vi "Build Delete.vi"(8 "error in (no error)":errorcluster, 9 "tableName":string, 10 "DynamicParameters in":refnum<class "DynamicParameters.lvclass">, 11 "DbConnection in":refnum<class "DbConnection.lvclass">) -> (0 "error out":errorcluster, 2 "Query":string, 3 "DbConnection out":refnum<class "DbConnection.lvclass">)   [LabVIEW 2020, in "ORM.lvlib" / "DbConnection.lvclass"]
uses:
  DbConnection.lvclass
  DynamicParameters/DynamicParameters.lvclass
  DbConnection.lvclass/DbConnection.ctl
  DynamicParameters/DynamicParameters.lvclass/DynamicParameters.ctl
  Read ColumnNameEqualsValueFormat.vi
  DynamicParameters/Read FieldNames.vi
  DynamicParameters/Read ParameterNames.vi
  DynamicParameters/Read KeyProperties.vi
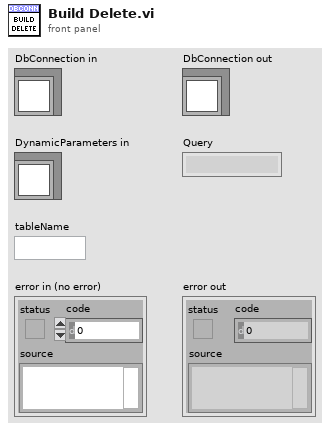
[diagram p1: front panel]
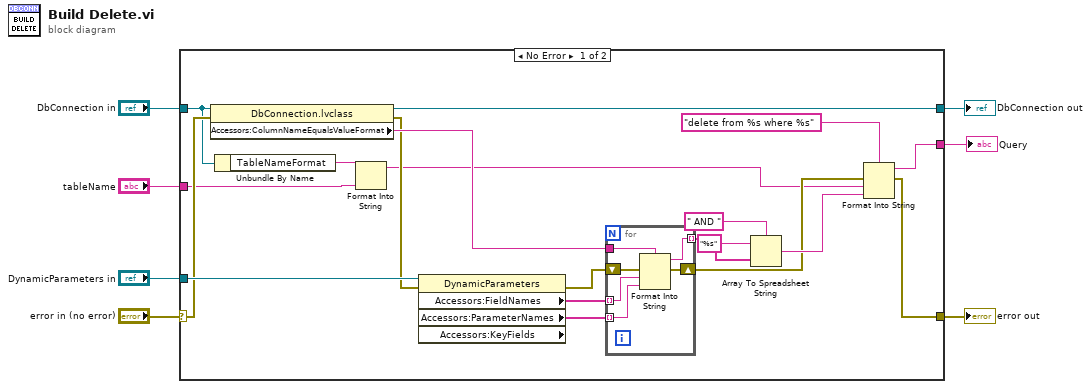
[diagram p0: block diagram]
diagram:
  n1 = case shown="No Error" "error in (no error)" {
    selector: "error in (no error)" -> [w18 w35]
    tunnel: [w14 w35] -> w6
    tunnel: [w27 w34] -> w4
    tunnel: "DbConnection in" -> [w11 w34]
    tunnel: "DynamicParameters in" -> [w26 _]
    tunnel: "tableName" -> [w9 _]
    tunnel: [w19 _] -> w1
    frame No Error {
      n2 = property class="DbConnection.lvclass"(reference=w11, error in=w18) -> (reference out=w27:refnum<class "DbConnection.lvclass">, error out=w17:errorcluster, "Accessors:ColumnNameEqualsValueFormat"=w23:string)
      n3 = Unbundle By Name(w11) -> ("TableNameFormat"=w10:string)
      n4 = Format Into String(format string=w10, w9) -> (resulting string=w8:string)  [unwired: 2 in, 1 out]
      n5 = property class="DynamicParameters" props=["Accessors:FieldNames", "Accessors:ParameterNames", "Accessors:KeyFields"](reference=w26, error in=w17) -> (error out=w16:errorcluster, "Accessors:FieldNames"=w25:string[], "Accessors:ParameterNames"=w24:string[])  [unwired: 2 out]
      n6 = for {
        tunnel: w25 -> [w29] mode=indexing
        tunnel: w24 -> [w32] mode=indexing
        tunnel: w23 -> [w33]
        tunnel: [w28] -> w20 mode=indexing
        shift-right: [w30] -> w15
        shift-left: w16 -> [w31]
        n7 = Format Into String(format string=w33, error in=w31, w29, w32) -> (resulting string=w28:string, error out=w30:errorcluster)  [unwired: 1 in]
      }
      n8 = Array To Spreadsheet String(delimiter (Tab)=" AND ", array=w20, 3:"%s" ("format string")) -> (spreadsheet string=w21:string)
      n9 = Format Into String(format string="delete from %s where %s", error in=w15, w8, w21) -> (resulting string=w19:string, error out=w14:errorcluster)  [unwired: 1 in]
    }
    frame Error {
    }
  }
  "error out" <- w6
  "DbConnection out" <- w4
  "Query" <- w1
